vi "Stop Process.vi"(8 "error in (no error)":errorcluster, 11 "Motor Controller in":refnum<class "Motor Controller.lvclass">) -> (0 "error out":errorcluster, 3 "Motor Controller out":refnum<class "Motor Controller.lvclass">)   [LabVIEW 2022 SP3, in "Motor Controller.lvclass"]
uses:
  Motor Controller.lvclass
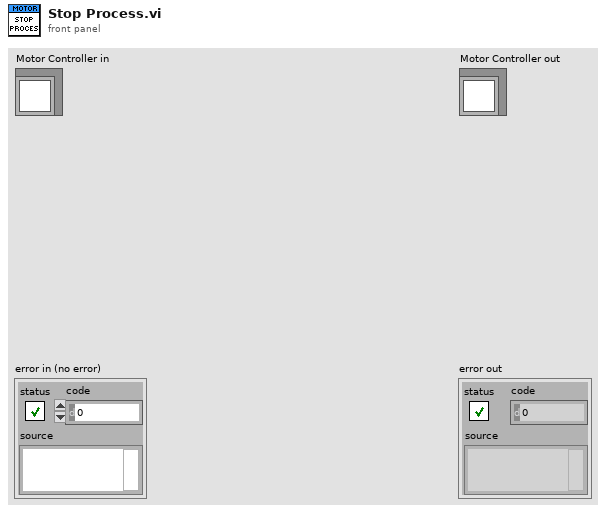
[diagram p1: front panel]
types:
  T1 = typedef "Motor Controller.lvclass/UserEvents.ctl" = cluster{"API Incoming Event":refnum<user-event>, "API Executed Event":refnum<user-event>, "API Return Event":refnum<user-event>, "Status Changed Event":refnum<user-event>, "StopEvent":refnum<user-event>}
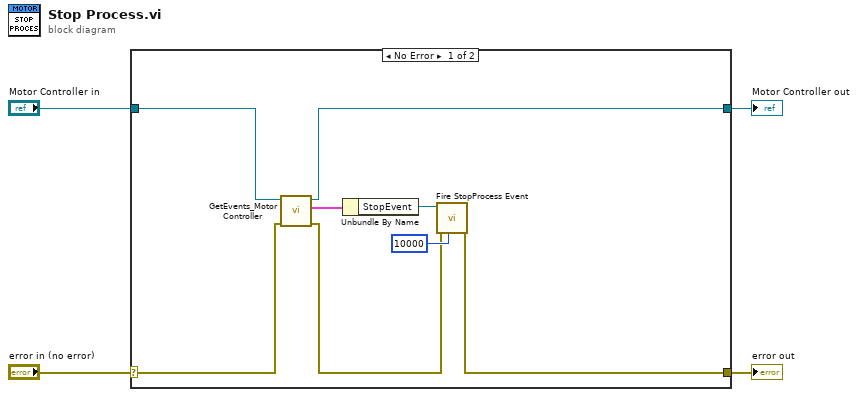
[diagram p0: block diagram]
diagram:
  n1 = case shown="No Error" "error in (no error)" {
    selector: "error in (no error)" -> [w7 w14]
    tunnel: [w5 w14] -> w3
    tunnel: [w12 w13] -> w1
    tunnel: "Motor Controller in" -> [w11 w13]
    frame No Error {
      n2 = call-dynamic "GetEvents_Motor Controller.vi"("error in (no error)"=w7, "TopLevel in"=w11) -> ("error out"=w6:errorcluster, "UserEvents"=w10:T1, "TopLevel out"=w12:refnum<class "Motor Controller.lvclass">)  [unwired: 7 in]
      n3 = Unbundle By Name(w10) -> ("StopEvent"=w9:refnum<user-event>)
      n4 = call "Fire StopProcess Event.vi"("timeout in ms (5000)"=10000, "error in (no error)"=w6, "Event in"=w9) -> ("error out"=w5:errorcluster)  [unwired: 5 in, 3 out]
    }
    frame Error {
    }
  }
  "error out" <- w3
  "Motor Controller out" <- w1
